vi "Disconnected.vi"(8 "error in (no error)":errorcluster, 10 "InstrumentData 2":T1, 11 "InterferometryUI in":refnum<class "InterferometryUI.lvclass">) -> (0 "error out":errorcluster, 3 "InterferometryUI out":refnum<class "InterferometryUI.lvclass">)   [LabVIEW 2023, in "InterferometryUI.lvlib" / "InterferometryUI.lvclass"]
uses:
  InterferometryUI.lvclass
  typedefs/instrumentType.ctl
  typedefs/typedefs.lvlib
  <vilib>/ActorFramework/Message Enqueuer/Message Enqueuer.lvclass
  typedefs/InstrumentData.ctl
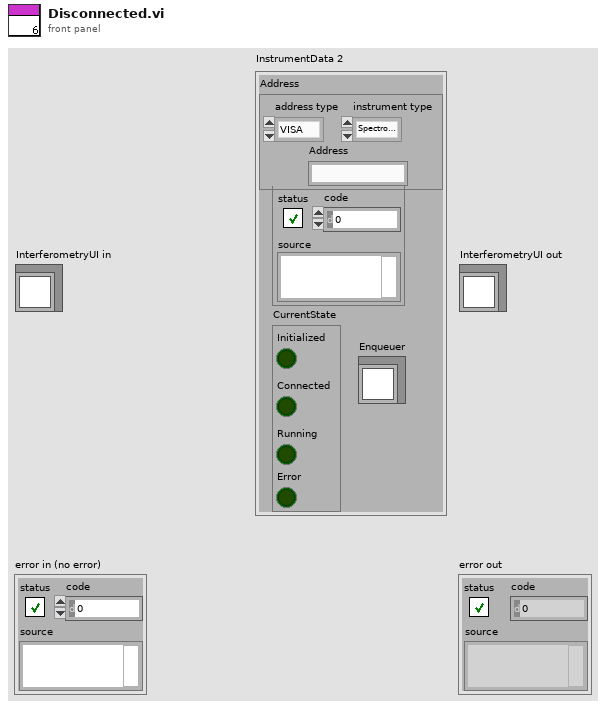
[diagram p1: front panel]
types:
  T1 = typedef "typedefs.lvlib/InstrumentData.ctl" = cluster{"Instr Error":errorcluster, "Address":cluster{"address type":enum16{"VISA", "Index"}, "Address":string, "instrument type":T2}, "CurrentState":cluster{"Initialized":bool, "Connected":bool, "Running":bool, "Error":bool}, "Enqueuer":refnum<class "Message Enqueuer.lvclass">}
  T2 = typedef "typedefs.lvlib/instrumentType.ctl" = enum16{"Spectrometer", "Camera", "Stepper"}
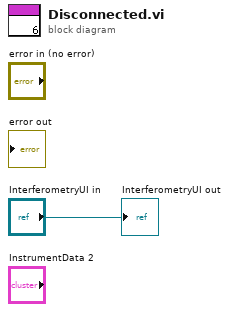
[diagram p0: block diagram]
diagram:
  "InterferometryUI out" <- "InterferometryUI in"
